vi "FPGA_Main_v01.vi"() -> ()   [LabVIEW 2014]
uses:
  <vilib>/rvi/Emulation/niFpgaGetClockAttributes.vi
  <vilib>/rvi/Emulation/niFpgaSctlEmulationGetInTimedLoop.vi
  <vilib>/rvi/Emulation/niFpgaEmulationReportErrorSimple.vi
  <vilib>/rvi/eio/common/nirviEmuTemplateMethod_errors.vi
  <vilib>/rvi/Emulation/niFpgaCriticalErrorInLSC.vi
  <vilib>/rvi/Emulation/niFpgaProcessEmulError.vi
  <vilib>/eio/EIONode/EIONode.xnode
panel:
  in  "Evac 3":bool
  in  "Evac 4":bool
  in  "Evac 1":bool
  in  "Evac 2":bool
  out "MFC N2-2":u8[](array[numeric])
  out "MFC O2":u8[](array[numeric])
  out "MFC N2":u8[](array[numeric])
  out "Valve Array In":fxp<+/-,30,9>[](array[numeric])
  in  "Valve Array Out":u8[](array[numeric])=[0, 0, 0, 0, 0, 0, 0, 0]
  in  "Emission SV 2":bool
  in  "Emission SV 1":bool
  in  "PR Test":bool
  out "MFC Error No.":u16
  out "MFC HC-2":u8[](array[numeric])
  out "MFC Air-2":u8[](array[numeric])
  out "MFC HC-B":u8[](array[numeric])
  out "MFC Array In":fxp<+/-,30,9>[](array[numeric])
  in  "MFC Array Out":u8[](array[numeric])=[65, 48, 48, 48, 48, 48, 13, 66, 48, 48, 48, 48, 48, 13, 67, 48, 48, 48, 48, 48, 13, 68, 48, 48, 48, 48, 48, 13, 70, 48, 48, 48, 48, 48, 13, 73, 48, 48, 48, 48, 48, 13, 74, 48, 48, 48, 48, 48, 13, 75, 48, 48, 48, 48, 48, 13, 76, 48, 48, 48, 48, 48, 13, 77, 48, 48, 48, 48, 48, 13, 78, 48, 48, 48, 48, 48, 13]
  in  "Furnace Array Out":u8[](array[numeric])=[65, 48, 48, 48, 48, 48, 13, 68, 48, 48, 48, 48]
  out "MFC Air-B":u8[](array[numeric])
  out "MFC NO":u8[](array[numeric])
  out "MFC AIR-1":u8[](array[numeric])
  out "MFC HC-1":u8[](array[numeric])
  out "MFC CO-1":u8[](array[numeric])
  in  "DO SV Array Out":bool[](array[boolean])=[FALSE, FALSE, FALSE, FALSE, FALSE, FALSE, FALSE, FALSE, FALSE, FALSE, FALSE, FALSE, FALSE]
  out "Array 1 In":fxp<+/-,35,9>[](array[numeric])
  in  "DO On?":bool
  in  "ISO1_SV":bool
  out "DI no 1":u16
  out "DI no 2":u8
  in  "TankHi":fxp<+/-,20,5>
  in  "TankLo":fxp<+/-,20,5>
  in  "Leak test on?":bool
  in  "Command":i16
  in  "Ramp rate,SP&CRC":u8[](array[numeric])=[66, 0, 0, 0, 132, 246]
  out "Active?":bool
  # "OMEGA FPGA v01"
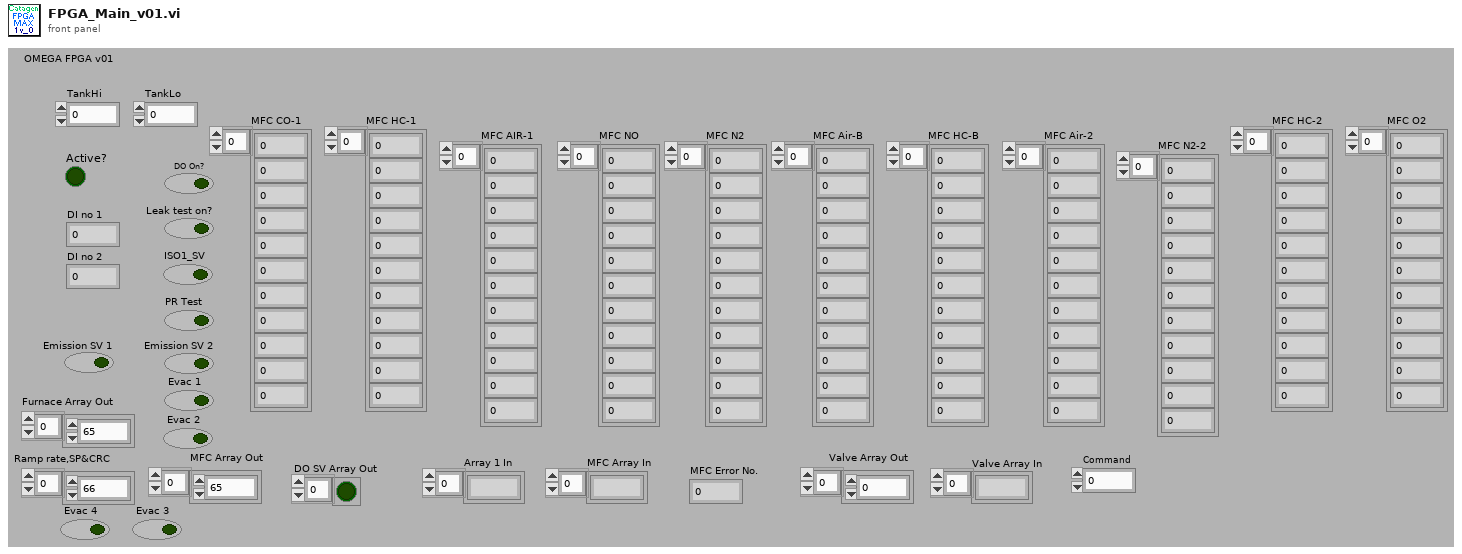
[diagram p1: front panel]
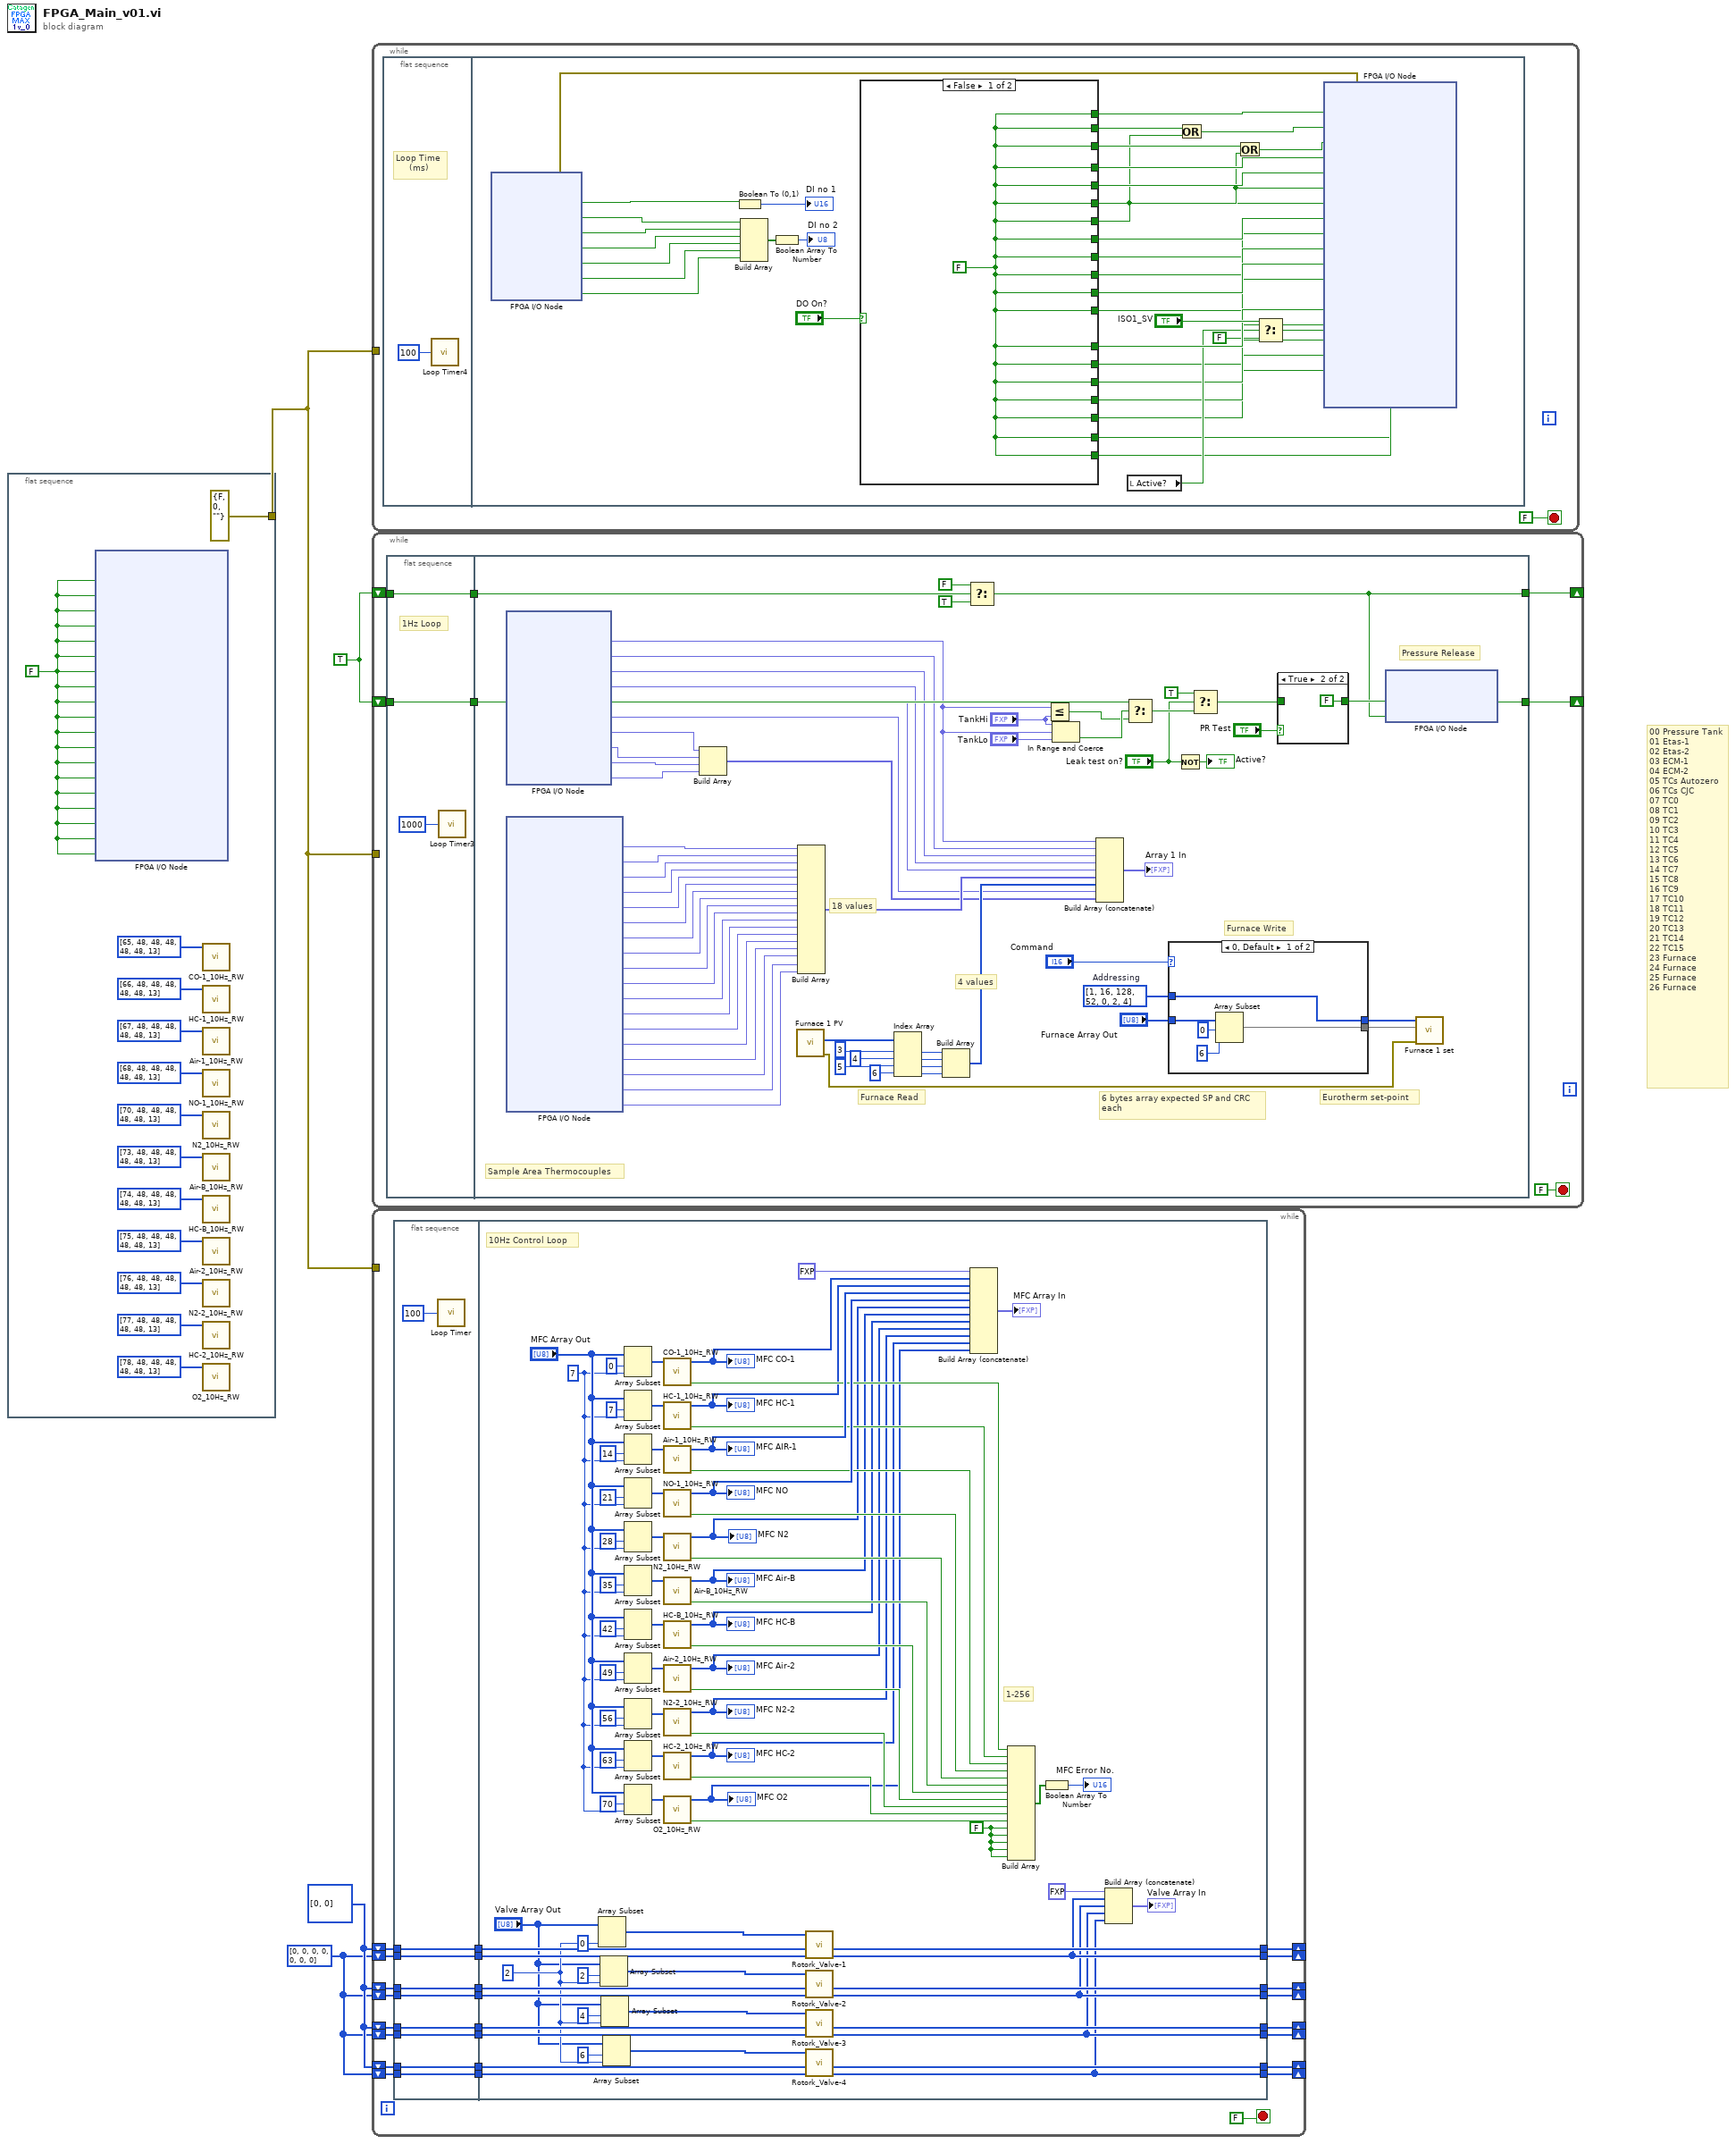
[diagram p0: block diagram]
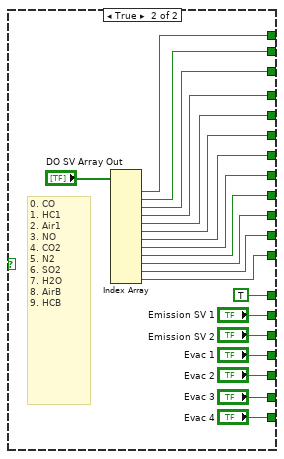
[diagram p2: hidden frame]
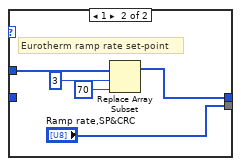
[diagram p4: hidden frame]
diagram:
  w2 = u8[] [0, 0, 0, 0, 0, 0, 0] ("Valve position")
  w3 = u8[] [0, 0] ("subarray")
  w1 = TRUE ("f")
  # "00 Pressure Tank\n01 Etas-1\n02 Etas-2\n03 ECM-1\n04 ECM-2\n05 TCs Autozero\n06 TCs CJC\n07 TC0\n08 TC1\n09 TC2\n10 TC3\n11 TC4\n12 TC5\n13 TC6\n14 TC7\n15 TC8\n16 TC9\n17 TC10\n18 TC11\n19 TC12\n20 TC13\n21 TC14\n22 TC15\n23 Furnace\n24 Furnace\n25 Furnace\n26 Furnace"
  n1 = flat-sequence {
    tunnel: [errorcluster {"status"=FALSE, "code"=0, "source"=""} ("error out")] -> w4
    frame #0 {
      w16 = FALSE
      n2 = xnode "FPGA I/O Node"("CO_SV"=w16, "HC-1_SV"=w16, "AIR-1_SV"=w16, "NO_SV"=w16, "CO2_SV"=w16, "N2-1_SV"=w16, "SO2_SV"=w16, "H2O_SV"=w16, "AIR-BAL_SV"=w16, "HC-BAL_SV"=w16, "AIR-2_SV"=w16, "N2-2_SV"=w16, "HC-2_SV"=w16, "O2_SV"=w16, "Tank-PR_SV"=w16, "Vent1_ISO1_SV"=w16, "Inverter_On"=w16, "Emission-1_ISO3_SV"=w16, "Emission-2_ISO4_SV"=w16) -> ()  [unwired: 20 in, 20 out]
      n3 = call "CO-1_10Hz_RW.vi"("Byte Array"=u8[] [65, 48, 48, 48, 48, 48, 13]) -> ()  [unwired: 9 in, 2 out]
      n4 = call "HC-1_10Hz_RW.vi"("Byte Array"=u8[] [66, 48, 48, 48, 48, 48, 13]) -> ()  [unwired: 9 in, 2 out]
      n5 = call "Air-1_10Hz_RW.vi"("Byte Array"=u8[] [67, 48, 48, 48, 48, 48, 13]) -> ()  [unwired: 9 in, 2 out]
      n6 = call "NO-1_10Hz_RW.vi"("Byte Array"=u8[] [68, 48, 48, 48, 48, 48, 13]) -> ()  [unwired: 9 in, 2 out]
      n7 = call "N2_10Hz_RW.vi"("Byte Array"=u8[] [70, 48, 48, 48, 48, 48, 13]) -> ()  [unwired: 9 in, 2 out]
      n8 = call "Air-B_10Hz_RW.vi"("Byte Array"=u8[] [73, 48, 48, 48, 48, 48, 13]) -> ()  [unwired: 9 in, 2 out]
      n9 = call "HC-B_10Hz_RW.vi"("Byte Array"=u8[] [74, 48, 48, 48, 48, 48, 13]) -> ()  [unwired: 9 in, 2 out]
      n10 = call "Air-2_10Hz_RW.vi"("Byte Array"=u8[] [75, 48, 48, 48, 48, 48, 13]) -> ()  [unwired: 9 in, 2 out]
      n11 = call "N2-2_10Hz_RW.vi"("Byte Array"=u8[] [76, 48, 48, 48, 48, 48, 13]) -> ()  [unwired: 9 in, 2 out]
      n12 = call "HC-2_10Hz_RW.vi"("Byte Array"=u8[] [77, 48, 48, 48, 48, 48, 13]) -> ()  [unwired: 9 in, 2 out]
      n13 = call "O2_10Hz_RW.vi"("Byte Array"=u8[] [78, 48, 48, 48, 48, 48, 13]) -> ()  [unwired: 9 in, 2 out]
    }
  }
  n14 = while {
    tunnel: w4 -> [_]
    stop <- FALSE stop-if-true
    n15 = flat-sequence {
      frame #0 {
        # "Loop Time\n     (ms)"
        n16 = call "Loop Timer4"("Count(mSec)"=u32 100) -> ()  [unwired: 1 out]
      }
      frame #1 {
        n17 = xnode "FPGA I/O Node"() -> ("error out"=w56:errorcluster, "eStop"=w23:bool, "Temp_SW1"=w53:bool, "Dr_1_Open"=w52:bool, "Dr_2_Open"=w51:bool, "Fan_On"=w41:bool, "Ext An Up"=w40:bool, "Ext An Dn"=w47:bool)  [unwired: 8 in, 7 out]
        n18 = Boolean To (0,1)(Boolean=w23) -> (0, 1=→"DI no 1":i16)
        n19 = Build Array(w53, w52, w51, w41, w40, w47) -> (w50:bool[])
        n20 = Boolean Array To Number(Boolean array=w50) -> (number=→"DI no 2":u8)
        n21 = case shown="False" "DO On?" {
          tunnel: [w57 w68] -> w43
          tunnel: [w57 w67] -> w29
          tunnel: [w57 w65] -> w42
          tunnel: [w57 w64] -> w26
          tunnel: [w57 TRUE] -> w48
          tunnel: [w57 w66] -> w32
          tunnel: [w57 w70] -> w28
          tunnel: [w57 w69] -> w27
          tunnel: [w57 w75] -> w39
          tunnel: [w57 w74] -> w33
          tunnel: [w57 w73] -> w31
          tunnel: [w57 w72] -> w38
          tunnel: [w57 w71] -> w37
          tunnel: [w57 "Emission SV 2"] -> w36
          tunnel: [w57 "Emission SV 1"] -> w35
          tunnel: [w57 "Evac 1"] -> w25
          tunnel: [w57 "Evac 2"] -> w24
          tunnel: [w57 "Evac 3"] -> w20
          tunnel: [w57 "Evac 4"] -> w21
          frame False {
            w57 = FALSE
          }
          frame True {
            # "0. CO\n1. HC1\n2. Air1\n3. NO\n4. CO2\n5. N2\n6. SO2\n7. H2O\n8. AirB\n9. HCB"
            n22 = Index Array(array="DO SV Array Out") -> (element #1=w75:bool, element #2=w74:bool, element #3=w73:bool, element #4=w72:bool, element #5=w71:bool, element #6=w70:bool, element #7=w69:bool, element #8=w68:bool, element #9=w67:bool, element #10=w66:bool, element #11=w65:bool, element #12=w64:bool)  [unwired: 12 in]
          }
        }
        n23 = local read "Active?"() -> (w44:bool)
        n24 = Or(x=w33, y=w27) -> (x .or. y?=w34:bool)
        n25 = Or(x=w31, y=w28) -> (x .or. y?=w30:bool)
        n26 = Select(t="ISO1_SV", s=w44, f=FALSE) -> (s? t:f=w45:bool)
        n27 = xnode "FPGA I/O Node"("error in"=w56, "CO_SV"=w39, "HC-1_SV"=w34, "AIR-1_SV"=w30, "NO_SV"=w38, "N2-1_SV"=w37, "AIR-BAL_SV"=w28, "HC-BAL_SV"=w27, "AIR-2_SV"=w43, "N2-2_SV"=w29, "HC-2_SV"=w32, "O2_SV"=w42, "HC_Switch_SV"=w26, "Vent1_ISO1_SV"=w45, "Inverter_On"=w48, "Emission-1_ISO3_SV"=w35, "Emission-2_ISO4_SV"=w36, "Evac-1 ISO6 SV"=w25, "Evac-2 ISO7 SV"=w24, "Evac-3"=w20, "Evac-4"=w21) -> ()  [unwired: 20 in, 21 out]
      }
    }
  }
  n28 = while {
    tunnel: w4 -> [_]
    shift-right: [w82] -> _
    shift-left: w1 -> [w83]
    shift-right: [w78] -> _
    shift-left: w1 -> [w79]
    stop <- FALSE ("stop") stop-if-true
    n29 = flat-sequence {
      tunnel: [w86] -> w81
      tunnel: w83 -> [w86]
      tunnel: [w85] -> w80
      tunnel: w79 -> [w85]
      tunnel: w81 -> [w150]
      tunnel: [w105] -> w82
      tunnel: w80 -> [w94]
      tunnel: [w93] -> w78
      frame #0 {
        # "1Hz Loop"
        n30 = call "Loop Timer3"("Count(mSec)"=u32 1000) -> ()  [unwired: 1 out]
      }
      frame #1 {
        w113 = u8[] [1, 16, 128, 52, 0, 2, 4]  # Addressing
        # "Pressure Release"
        # "Furnace Write"
        # "Furnace Read"
        # "Sample Area Thermocouples"
        # "4 values"
        # "18 values"
        # "6 bytes array expected SP and CRC\neach"
        # "Eurotherm set-point"
        n31 = xnode "FPGA I/O Node"() -> ("Pressure_Tank"=w102:fxp<+/-,26,5>, "Etas-1"=w101:fxp<+/-,26,5>, "Etas-2"=w100:fxp<+/-,26,5>, "ECM-1"=w99:fxp<+/-,26,5>, "ECM-2"=w98:fxp<+/-,26,5>, "Furnace In"=w97:fxp<+/-,26,5>, "PT-1"=w91:fxp<+/-,26,5>, "PT-2"=w90:fxp<+/-,26,5>, "PT-3"=w89:fxp<+/-,26,5>, "PT-4"=w88:fxp<+/-,26,5>)  [unwired: 11 in, 11 out]
        n32 = xnode "FPGA I/O Node"() -> ("04 TCs/Autozero"=w146:fxp<+/-,24,-2>, "04 TCs/CJC"=w147:fxp<+/-,24,-2>, "04 TCs/TC0"=w119:fxp<+/-,24,-2>, "04 TCs/TC1"=w120:fxp<+/-,24,-2>, "04 TCs/TC2"=w121:fxp<+/-,24,-2>, "04 TCs/TC3"=w122:fxp<+/-,24,-2>, "04 TCs/TC4"=w123:fxp<+/-,24,-2>, "04 TCs/TC5"=w124:fxp<+/-,24,-2>, "04 TCs/TC6"=w125:fxp<+/-,24,-2>, "04 TCs/TC7"=w126:fxp<+/-,24,-2>, "04 TCs/TC8"=w127:fxp<+/-,24,-2>, "04 TCs/TC9"=w111:fxp<+/-,24,-2>, "04 TCs/TC10"=w109:fxp<+/-,24,-2>, "04 TCs/TC11"=w110:fxp<+/-,24,-2>, "04 TCs/TC12"=w108:fxp<+/-,24,-2>, "04 TCs/TC13"=w107:fxp<+/-,24,-2>, "04 TCs/TC14"=w128:fxp<+/-,24,-2>, "04 TCs/TC15"=w129:fxp<+/-,24,-2>)  [unwired: 19 in, 19 out]
        n33 = Build Array(w91, w90, w89, w88) -> (w92:fxp<+/-,26,5>[])
        n34 = call "Furnace 1 PV.vi"() -> ("error out"=w114:errorcluster, "Array"=w145:u8[])  [unwired: 10 in]
        n35 = Build Array(w146, w147, w119, w120, w121, w122, w123, w124, w125, w126, w127, w111, w109, w110, w108, w107, w128, w129) -> (w117:fxp<+/-,24,-2>[])
        n36 = Index Array(array=w145, index #1=3, index #2=4, index #3=5, index #4=6 ("index")) -> (element #1=w137:u8, element #2=w138:u8, element #3=w139:u8, element #4=w140:u8)
        n37 = Build Array(w137, w138, w139, w140) -> (w118:u8[])
        n38 = Select(t=FALSE, s=w94, f=TRUE) -> (s? t:f=w93:bool)
        n39 = Less Or Equal?(x=w102, y="TankHi") -> (x <= y?=w103:bool)
        n40 = In Range and Coerce(upper limit="TankHi", x=w102, lower limit="TankLo") -> (In Range?=w136:bool)  [unwired: 1 out]
        n41 = Build Array (concatenate)(w102, w101, w100, w99, w98, w117, w118, w97, w92) -> (→"Array 1 In":fxp<+/-,35,9>[])
        n42 = Select(t=w150, s=w136, f=w103) -> (s? t:f=w133:bool)
        n43 = case shown="0, Default" "Command" {
          tunnel: [w154 w160] -> w115
          tunnel: "Furnace Array Out" -> [w155 _]
          tunnel: [w153 "Ramp rate,SP&CRC"] -> w148
          tunnel: w113 -> [w154 w161]
          frame 0, Default {
            n44 = Array Subset(array=w155, index=0, length=6) -> (w153:u8[])
          }
          frame 1 {
            # "Eurotherm ramp rate set-point"
            n45 = Replace Array Subset(array=w161, new element=u8 70 ("new element/subarray"), index=3) -> (w160:u8[])
          }
        }
        n46 = Not(x="Leak test on?") -> (.not. x?=→"Active?":bool)
        n47 = Select(t=TRUE, s="Leak test on?", f=w133) -> (s? t:f=w106:bool)
        n48 = case shown="True" "PR Test" {
          tunnel: w106 -> [w151 _]
          tunnel: [w151 FALSE ("f")] -> w105
          frame False {
          }
          frame True {
          }
        }
        n49 = xnode "FPGA I/O Node"("Tank-PR_SV"=w105, "USER FPGA LED"=w93) -> ()  [unwired: 3 in, 3 out]
        n50 = call "Furnace 1 set.vi"("error in"=w114, "SP&CRC"=w148, "Addressing"=w115) -> ()  [unwired: 8 in, 1 out]
      }
    }
  }
  n51 = while {
    tunnel: w4 -> [_]
    shift-right: [w186] -> _
    shift-left: w3 -> [w184]
    shift-right: [w183] -> _
    shift-left: w2 -> [w181]
    shift-right: [w180] -> _
    shift-left: w3 -> [w172]
    shift-right: [w179] -> _
    shift-left: w2 -> [w171]
    shift-right: [w170] -> _
    shift-left: w3 -> [w168]
    shift-right: [w169] -> _
    shift-left: w2 -> [w167]
    shift-right: [w166] -> _
    shift-left: w3 -> [w164]
    shift-right: [w165] -> _
    shift-left: w2 -> [w163]
    stop <- FALSE stop-if-true
    n52 = flat-sequence {
      tunnel: [w195] -> w185
      tunnel: w184 -> [w195]
      tunnel: [w194] -> w182
      tunnel: w181 -> [w194]
      tunnel: w172 -> [w193]
      tunnel: [w193] -> w178
      tunnel: w171 -> [w192]
      tunnel: [w192] -> w177
      tunnel: w168 -> [w191]
      tunnel: [w191] -> w176
      tunnel: w167 -> [w190]
      tunnel: [w190] -> w175
      tunnel: w164 -> [w189]
      tunnel: [w189] -> w174
      tunnel: w163 -> [w188]
      tunnel: [w188] -> w173
      tunnel: [w251] -> w186
      tunnel: w185 -> [w253]
      tunnel: [w232] -> w183
      tunnel: w182 -> [w252]
      tunnel: [w249] -> w180
      tunnel: [w231] -> w179
      tunnel: w178 -> [w248]
      tunnel: w177 -> [w247]
      tunnel: w176 -> [w246]
      tunnel: w175 -> [w245]
      tunnel: w174 -> [w244]
      tunnel: w173 -> [w243]
      tunnel: [w242] -> w170
      tunnel: [w230] -> w169
      tunnel: [w241] -> w166
      tunnel: [w229] -> w165
      frame #0 {
        n53 = call "Loop Timer"("Count(mSec)"=u32 100) -> ()  [unwired: 1 out]
      }
      frame #1 {
        w197 = FALSE ("element")
        (unwired) 0 ("length")
        w239 = 2 ("length")
        w219 = 7 ("length")
        # "1-256"
        # "10Hz Control Loop"
        n54 = Array Subset(array="Valve Array Out", length=w239) -> (w250:u8[])  [unwired: 1 in]
        n55 = Array Subset(array="Valve Array Out", index=2, length=w239) -> (w240:u8[])
        n56 = Array Subset(array="Valve Array Out", index=4, length=w239) -> (w233:u8[])
        n57 = Array Subset(array="Valve Array Out", index=6, length=w239) -> (w234:u8[])
        n58 = Array Subset(array="MFC Array Out", index=0, length=w219) -> (w264:u8[])
        n59 = Array Subset(array="MFC Array Out", index=7, length=w219) -> (w263:u8[])
        n60 = Array Subset(array="MFC Array Out", index=14, length=w219) -> (w262:u8[])
        n61 = Array Subset(array="MFC Array Out", index=21, length=w219) -> (w261:u8[])
        n62 = Array Subset(array="MFC Array Out", index=28, length=w219) -> (w224:u8[])
        n63 = Array Subset(array="MFC Array Out", index=35, length=w219) -> (w260:u8[])
        n64 = Array Subset(array="MFC Array Out", index=42, length=w219) -> (w259:u8[])
        n65 = Array Subset(array="MFC Array Out", index=49, length=w219) -> (w258:u8[])
        n66 = Array Subset(array="MFC Array Out", index=56, length=w219) -> (w222:u8[])
        n67 = Array Subset(array="MFC Array Out", index=63, length=w219) -> (w257:u8[])
        n68 = Array Subset(array="MFC Array Out", index=70, length=w219) -> (w218:u8[])
        n69 = call "CO-1_10Hz_RW.vi"("Byte Array"=w264) -> ("Fault"=w217:bool, "MFC out"=w201:u8[])  [unwired: 9 in]
        "MFC CO-1" <- w201
        n70 = call "HC-1_10Hz_RW.vi"("Byte Array"=w263) -> ("Fault"=w216:bool, "MFC out"=w202:u8[])  [unwired: 9 in]
        "MFC HC-1" <- w202
        n71 = call "Air-1_10Hz_RW.vi"("Byte Array"=w262) -> ("Fault"=w215:bool, "MFC out"=w256:u8[])  [unwired: 9 in]
        "MFC AIR-1" <- w256
        n72 = call "NO-1_10Hz_RW.vi"("Byte Array"=w261) -> ("Fault"=w214:bool, "MFC out"=w255:u8[])  [unwired: 9 in]
        "MFC NO" <- w255
        n73 = call "N2_10Hz_RW.vi"("Byte Array"=w224) -> ("Fault"=w213:bool, "MFC out"=w199:u8[])  [unwired: 9 in]
        "MFC N2" <- w199
        n74 = call "Air-B_10Hz_RW.vi"("Byte Array"=w260) -> ("Fault"=w212:bool, "MFC out"=w206:u8[])  [unwired: 9 in]
        "MFC Air-B" <- w206
        n75 = call "HC-B_10Hz_RW.vi"("Byte Array"=w259) -> ("Fault"=w211:bool, "MFC out"=w205:u8[])  [unwired: 9 in]
        "MFC HC-B" <- w205
        n76 = call "Air-2_10Hz_RW.vi"("Byte Array"=w258) -> ("Fault"=w210:bool, "MFC out"=w204:u8[])  [unwired: 9 in]
        "MFC Air-2" <- w204
        n77 = call "N2-2_10Hz_RW.vi"("Byte Array"=w222) -> ("Fault"=w209:bool, "MFC out"=w198:u8[])  [unwired: 9 in]
        "MFC N2-2" <- w198
        n78 = call "HC-2_10Hz_RW.vi"("Byte Array"=w257) -> ("Fault"=w208:bool, "MFC out"=w203:u8[])  [unwired: 9 in]
        "MFC HC-2" <- w203
        n79 = call "O2_10Hz_RW.vi"("Byte Array"=w218) -> ("Fault"=w207:bool, "MFC out"=w200:u8[])  [unwired: 9 in]
        "MFC O2" <- w200
        n80 = call "Rotork_Valve-1.vi"("Array In 2"=w252, "Array In 1"=w253, "Valve SP"=w250) -> ("Array Out 2"=w232:u8[], "Array Out 1"=w251:u8[])  [unwired: 7 in]
        n81 = call "Rotork_Valve-2.vi"("Array In 2"=w247, "Array In 1"=w248, "Valve SP"=w240) -> ("Array Out 2"=w231:u8[], "Array Out 1"=w249:u8[])  [unwired: 7 in]
        n82 = call "Rotork_Valve-3.vi"("Array In 2"=w245, "Array In 1"=w246, "Valve SP"=w233) -> ("Array Out 2"=w230:u8[], "Array Out 1"=w242:u8[])  [unwired: 7 in]
        n83 = call "Rotork_Valve-4.vi"("Array In 2"=w243, "Array In 1"=w244, "Valve SP"=w234) -> ("Array Out 2"=w229:u8[], "Array Out 1"=w241:u8[])  [unwired: 7 in]
        n84 = Build Array (concatenate)(fxp<+/-,26,5> 0.0 ("Pressure_Tank"), w201, w202, w256, w255, w199, w206, w205, w204, w198, w203, w200) -> (→"MFC Array In":fxp<+/-,30,9>[])
        n85 = Build Array(w217, w216, w215, w214, w213, w212, w211, w210, w209, w208, w207, w197, w197, w197, w197, w197) -> (w266:bool[])
        n86 = Boolean Array To Number(Boolean array=w266) -> (number=→"MFC Error No.":u16)
        n87 = Build Array (concatenate)(fxp<+/-,26,5> 0.0 ("Pressure_Tank"), w232, w231, w230, w229) -> (→"Valve Array In":fxp<+/-,30,9>[])
      }
    }
  }
